vi "Get Background.vi"(8 "error in (no error)":errorcluster, 10 "size":u32, 11 "arr":i32) -> (0 "error out":errorcluster, 2 "function return":u32, 3 "arr out":i32)   [LabVIEW 2014, in "atmcd32d.lvlib"]
doc: "unsigned int WINAPI GetBackground(at_32 * arr, unsigned long size);"
uses:
  atmcd32d.lvlib
  atmcd32d.dll
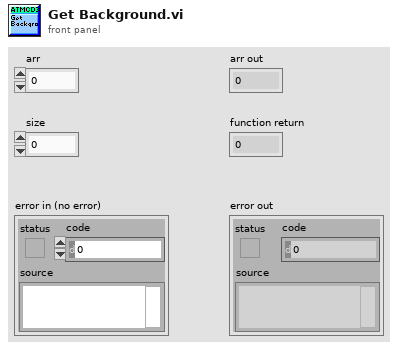
[diagram p1: front panel]
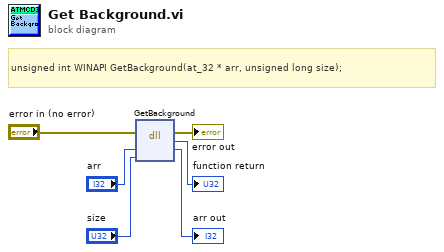
[diagram p0: block diagram]
diagram:
  # "unsigned int WINAPI GetBackground(at_32 * arr, unsigned long size);"
  n1 = dll-call lib="C:/Users/Bakir/Documents/Lambda2-Testing/lib/Andorlib/atmcd32d.*" fn="GetBackground"(error in="error in (no error)", "arr"="arr", "size"="size") -> (error out=→"error out":errorcluster, →"function return":u32, "arr"=→"arr out":i32)  [unwired: 3 in, 1 out]
